vi "TCP Write Stream.vi"(5 "file dialog info":T1={"prompt"="Please select a file to read from", "pattern"="*", "default name"="", "start path"=path ""}, 6 "chunk size (4096)":i32=4096, 7 "binary":bool=TRUE, 8 "error in (no error)":errorcluster, 9 "data":string, 10 "data file (<NAP>)":path=path "", 11 "connection":refnum<k5>) -> (0 "error out":errorcluster, 1 "bytes written":i32, 2 "data file out":path, 3 "duplicate connection":refnum<k5>, 4 "file error":errorcluster)   [LabVIEW 2017, in "NI_FTP.lvlib"]
doc: "Write all data to a TCP.\nIf \"data file\" is specified, its contents are written, otherwise \"data\" is used.\nIf \"binary\" is FALSE, EOLN characters in the data will be replaced with CRLF..\n\"chunk size\" determines how many bytes at a time are read from the file"
uses:
  <vilib>/FTP/NI_FTP.lvlib
panel:
  in  "(no error)":errorcluster
  in  "refnum":refnum<file>
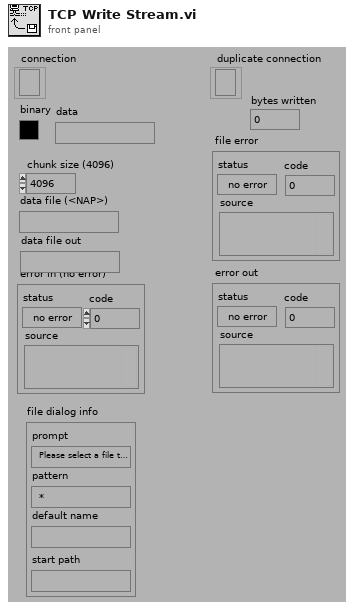
[diagram p1: front panel]
types:
  T1 = cluster{"prompt":string, "pattern":string, "default name":string, "start path":path}
  T2 = enum16{"read/write", "read-only", "write-only", "write-only (truncate)"}
  T3 = enum16{"open", "open or create", "create or replace", "create"}
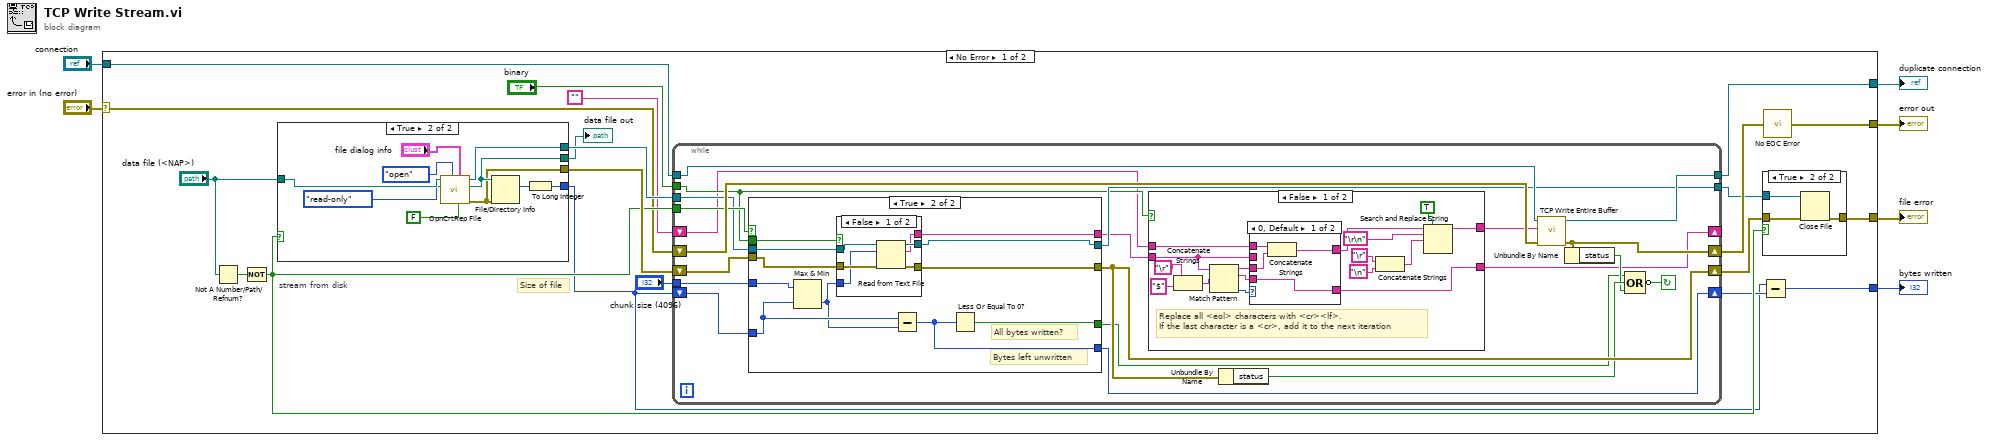
[diagram p0: block diagram]
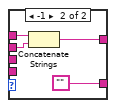
[diagram p2: hidden frame]
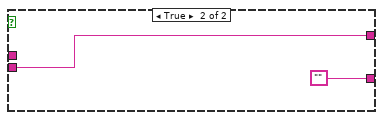
[diagram p3: hidden frame]
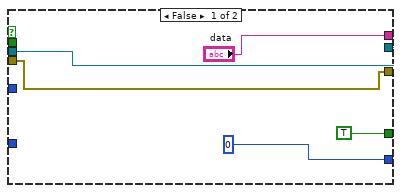
[diagram p4: hidden frame]
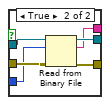
[diagram p5: hidden frame]
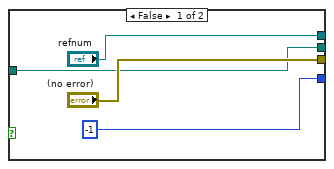
[diagram p7: hidden frame]
diagram:
  n1 = case shown="No Error" "error in (no error)" {
    selector: "error in (no error)" -> [w8 w120]
    tunnel: [w21 w120] -> w6
    tunnel: [w20 w121] -> w5
    tunnel: [w16 _] -> w4
    tunnel: [w11 _] -> w3
    tunnel: "connection" -> [w10 w121]
    frame No Error {
      # "Size of file"
      # "stream from disk"
      n2 = Not A Number/Path/Refnum?(number/path/refnum="data file (<NAP>)") -> (NaN/Path/Refnum?=w23:bool)
      n3 = Not(x=w23) -> (.not. x?=w19:bool)
      n4 = case shown="True" w19 {
        tunnel: "data file (<NAP>)" -> [w106 w119]
        tunnel: ["refnum" w116] -> w25
        tunnel: ["(no error)" w115] -> w24
        tunnel: [-1 ("size") w114] -> w12
        tunnel: [w106 w117] -> w14
        frame False {
        }
        frame True {
          n5 = call <vilib>:"OpnCrtRep File.vi"("advisory dialog? (display:T)"=FALSE, "file dialog info"="file dialog info", "function (open:0)"=T3."open", "open mode (0)"=T2."read-only", "file path"=w119) -> ("error out"=w115:errorcluster, "new file path"=w117:path, "refnum"=w116:refnum<file>)  [unwired: 3 in, 1 out]
          n6 = File/Directory Info(path=w117, error in=w115) -> (size=w110:i64)  [unwired: 6 out]
          n7 = To Long Integer(number=w110) -> (32bit integer=w114:i32)
        }
      }
      "data file out" <- w14
      n8 = while {
        shift-left: w12 -> [w34]
        shift-right: [w33] -> w15
        tunnel: [w37] -> w17
        tunnel: [w42] -> w20
        tunnel: w10 -> [w43]
        tunnel: "binary" -> [w32]
        tunnel: w19 -> [w46]
        shift-left: w8 -> [w47]
        shift-right: [w35] -> w22
        shift-left: w24 -> [w45]
        shift-right: [w41] -> w18
        tunnel: w25 -> [w44]
        shift-right: [w29] -> _
        shift-left: "" -> [w30]
        tunnel: "chunk size (4096)" -> [w27]
        stop <- w38 continue-if-true
        n9 = case shown="True" w46 {
          tunnel: w45 -> [w78 w88]
          tunnel: [w78 w82] -> w41
          tunnel: w32 -> [_ w89]
          tunnel: w44 -> [w77 w85]
          tunnel: [w77 w83] -> w37
          tunnel: ["data" w84] -> w31
          tunnel: [TRUE w80] -> w36
          tunnel: w34 -> [_ w87]
          tunnel: [0 w81] -> w33
          tunnel: w27 -> [_ w79]
          frame False {
          }
          frame True {
            # "All bytes written?"
            # "Bytes left unwritten"
            n10 = Max & Min(x=w79, y=w87) -> (min(x,y)=w86:i32)  [unwired: 1 out]
            n11 = case shown="False" w89 {
              tunnel: [w94 w101] -> w82
              tunnel: w88 -> [w95 w100]
              tunnel: w86 -> [w91 w99]
              tunnel: w85 -> [w92 w98]
              tunnel: [w93 w97] -> w83
              tunnel: [w90 w96] -> w84
              frame False {
                n12 = Read from Text File(file (use dialog)=w92, count=w91, error in=w95) -> (refnum out=w93:refnum<file>, text=w90:string, error out=w94:errorcluster)  [unwired: 2 out]
              }
              frame True {
                n13 = Read from Binary File(8:w100, 10:w99, 11:w98) -> (0:w101:errorcluster, 2:w96:string, 3:w97:refnum<file>)  [unwired: 4 out]
              }
            }
            n14 = Subtract(x=w87, y=w86) -> (x-y=w81:i32)
            n15 = Less Or Equal To 0?(x=w81) -> (x <= 0?=w80:bool)
          }
        }
        n16 = case shown="False" w32 {
          tunnel: w31 -> [w60 w72]
          tunnel: w30 -> [w59 _]
          tunnel: [w58 ""] -> w29
          tunnel: [w51 w72] -> w28
          frame False {
            # "Replace all <eol> characters with <cr><lf>.\nIf the last character is a <cr>, add it to the next iteration"
            n17 = Concatenate Strings("\r", "$" ("string")) -> (w50:string)
            n18 = Match Pattern(string=w60, regular expression=w50) -> (before substring=w62:string, match substring=w63:string, offset past match=w61:i32)  [unwired: 2 out]
            n19 = case shown="0, Default" w61 {
              tunnel: w59 -> [w67 w70]
              tunnel: [w64 ""] -> w58
              tunnel: w60 -> [_ w69]
              tunnel: [w65 w68] -> w57
              tunnel: w62 -> [w66 _]
              tunnel: w63 -> [w64 _]
              frame 0, Default {
                n20 = Concatenate Strings(w67, w66) -> (w65:string)
              }
              frame -1 {
                n21 = Concatenate Strings(w70, w69) -> (w68:string)
              }
            }
            n22 = Concatenate Strings("\r", "\n") -> (w52:string)
            n23 = Search and Replace String(replace all?=TRUE ("replace all? (F)"), input string=w57, search string="\r\n", replace string=w52) -> (result string=w51:string)  [unwired: 1 in, 6 out]
          }
          frame True {
          }
        }
        n24 = Unbundle By Name(w41) -> ("status"=w40:bool)
        n25 = call <vilib>:"TCP Write Entire Buffer.vi"("error in (no error)"=w47, "data in"=w28, "connection ID"=w43) -> ("error out"=w35:errorcluster, "connection ID out"=w42:refnum<k5>)  [unwired: 7 out]
        n26 = Unbundle By Name(w35) -> ("status"=w39:bool)
        n27 = Compound Arithmetic op=OR(w36, w40, w39) -> (invert w38:bool)
      }
      n28 = Subtract(x=w12, y=w15) -> (x-y=w11:i32)
      n29 = case shown="True" w19 {
        tunnel: w18 -> [w102 w105]
        tunnel: w17 -> [_ w104]
        tunnel: [w102 w103] -> w16
        frame False {
        }
        frame True {
          n30 = Close File(refnum=w104, error in=w105) -> (error out=w103:errorcluster)  [unwired: 1 out]
        }
      }
      n31 = call <vilib>:"No EOC Error.vi"("error in (no error)"=w22) -> ("error out"=w21:errorcluster)  [unwired: 4 out]
    }
    frame Error {
    }
  }
  "error out" <- w6
  "duplicate connection" <- w5
  "file error" <- w4
  "bytes written" <- w3
